vi "10-03-22.vi"() -> ()   [LabVIEW 2015]
uses:
  <vilib>/userdefined/High Color/IMAQdx.ctl
  <vilib>/vision/NI_Vision_Development_Module.lvlib
  <vilib>/vision/driver/NI_Vision_Acquisition_Software.lvlib
panel:
  out "Image 2":T1(plugin-control)
  in  "BCG Values":T2={"Brightness"=171.0, "Contrast"=56.0, "Gamma"=2.0} {"Gamma" min=0.1 max=10 step=0.01 scale=10.0..0.1; "Contrast" min=1 max=89 step=1 scale=30.0..89.0; "Brightness" min=0 max=255 step=1 scale=0.0..255.0}
  out "Processed Image":T1(plugin-control)
  out "error out":errorcluster
  in  "Image Type 2":T3 items=["Grayscale (U8)", "Grayscale (I16)", "Grayscale (SGL)", "Complex (CSG)", "RGB (U32)", "HSL (U32)", "RGB (U64)", "Grayscale (U16)"]
  out "error out 3":errorcluster
  in  "Session In 2":T4
  out "Quantity":i32
  out "Tong K/lg (kg)":dbl
  out "Mass (kg):":dbl
  out "Style":string
  out "Data":string
  out "Found?":bool
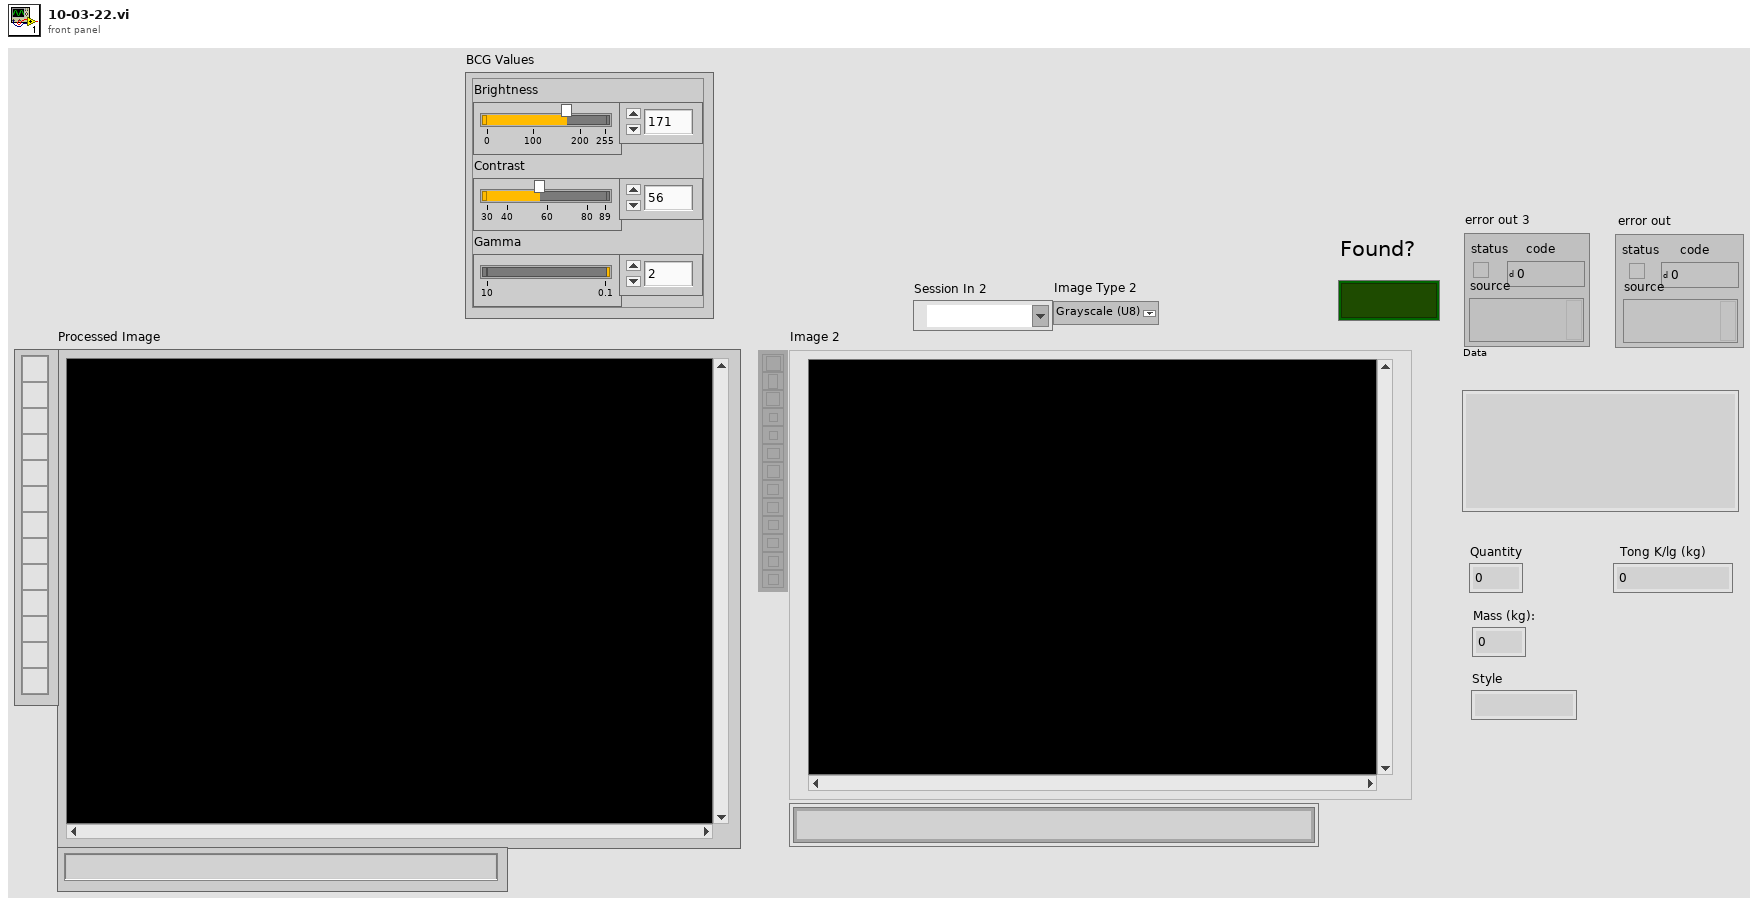
[diagram p1: front panel]
types:
  T1 = typedef "IMAQ Image.ctl" = refnum<image>
  T2 = cluster{"Brightness":sgl, "Contrast":sgl, "Gamma":sgl}
  T3 = typedef "Image Type" = u32
  T4 = typedef "IMAQdx.ctl" = refnum<k21>
  T5 = typedef "QR Code Report.ctl" = cluster{"Found?":bool, "Data":string, "Bounding Box":cluster{"x":sgl, "y":sgl}[], "Errors Corrected":u32, "Dimensions (Rows/Cols)":u32, "Version":u32, "QR Model":T6, "Stream Mode":T7, "Barcode Polarity":T8, "Mirrored?":bool, "Append Stream Position":u32, "Size of Append Stream":u32, "First EAN-128 ID":i32, "First Alternate Language ID":i32, "Append Stream ID":u32, "Minimum Edge Strength":u32, "Demodulation Mode":T9, "Cell Sample Size":T10, "Cell Filter Mode":T11}
  T6 = typedef "QR Code Model Type.ctl" = i32
  T7 = typedef "QR Code Stream Mode Type.ctl" = i32
  T8 = typedef "Data Matrix Polarity.ctl" = i32
  T9 = typedef "Demodulation Mode.ctl" = i32
  T10 = typedef "Cell Sample Size.ctl" = i32
  T11 = typedef "Cell Filter Mode.ctl" = i32
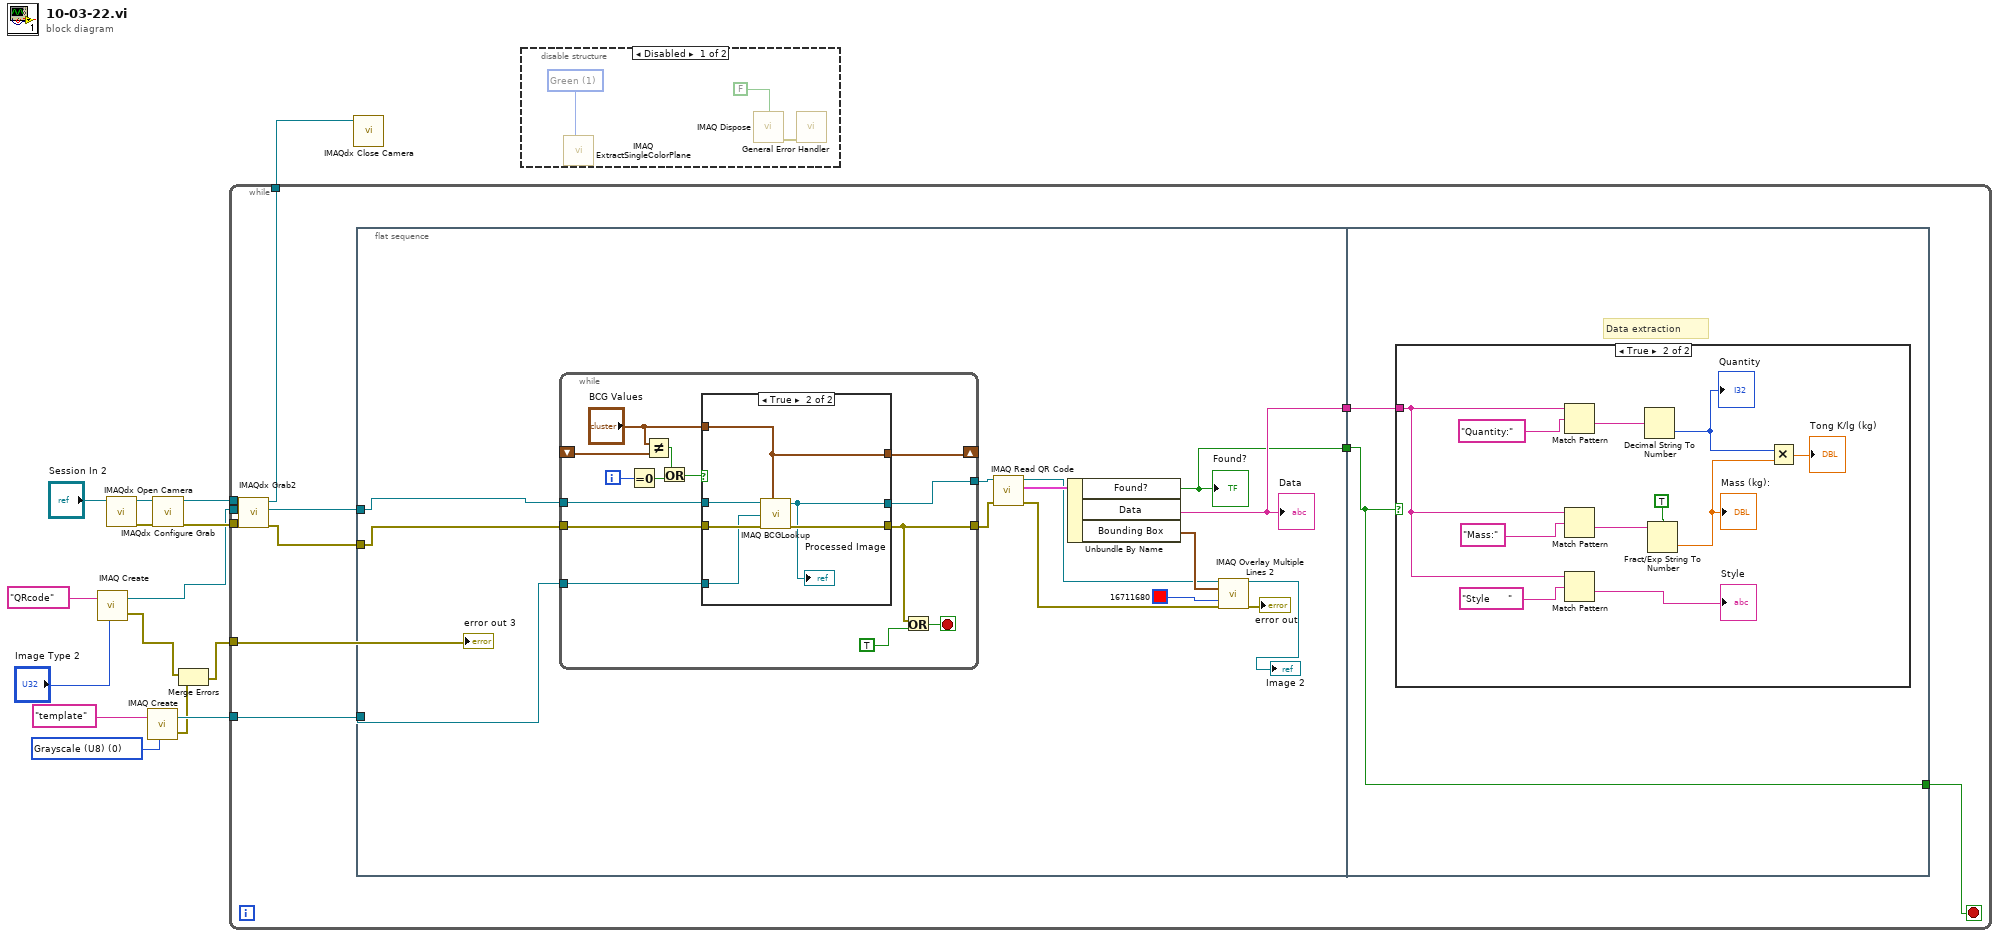
[diagram p0: block diagram]
diagram:
  w9 = T3 0 items=["Grayscale (U8)", "Grayscale (I16)", "Grayscale (SGL)", "Complex (CSG)", "RGB (U32)", "HSL (U32)", "RGB (U64)", "Grayscale (U16)"] ("Image Type")
  n1 = call "IMAQ Create"("Image Name"="QRcode", "Image Type"="Image Type 2") -> ("New Image"=w2:T1, "error out"=w7:errorcluster)  [unwired: 3 in]
  n2 = call <vilib>:"IMAQdx Open Camera.vi"("Session In"="Session In 2") -> ("error out"=w11:errorcluster, "Session Out"=w14:T4)  [unwired: 9 in]
  n3 = call "IMAQ Create"("Image Name"="template", "Image Type"=w9) -> ("New Image"=w8:T1, "error out"=w6:errorcluster)  [unwired: 3 in]
  n4 = call <vilib>:"IMAQdx Configure Grab.vi"("error in"=w11, "Session In"=w14) -> ("error out"=w3:errorcluster, "Session Out"=w4:T4)  [unwired: 8 in]
  n5 = Merge Errors(w7, w6) -> (w5:errorcluster)
  n6 = while {
    tunnel: w8 -> [w24]
    tunnel: w5 -> [w23]
    tunnel: w4 -> [w22]
    tunnel: w3 -> [w21]
    tunnel: w2 -> [w19]
    tunnel: [w16] -> w1
    stop <- w17 stop-if-true
    n7 = call <vilib>:"IMAQdx Grab2.vi"("error in"=w21, "Image In"=w19, "Session In"=w22) -> ("error out"=w20:errorcluster, "Image Out"=w18:T1, "Session Out"=w16:T4)  [unwired: 5 in, 1 out]
    n8 = flat-sequence {
      tunnel: [w36] -> w26
      tunnel: [w30] -> w25
      tunnel: w24 -> [w33]
      tunnel: w20 -> [w27]
      tunnel: w18 -> [w28]
      tunnel: w26 -> [w65]
      tunnel: w25 -> [w64]
      tunnel: [w64] -> w17
      frame #0 {
        n9 = while {
          tunnel: w27 -> [w54]
          tunnel: w28 -> [w53]
          tunnel: w33 -> [w52]
          shift-right: [w51] -> _
          shift-left: _ -> [w50]
          tunnel: [w44] -> w32
          tunnel: [w41] -> w34
          i -> [w48]
          stop <- w43 stop-if-true
          n10 = Equal To 0?(x=w48) -> (x = 0?=w46:bool)
          n11 = Not Equal?(x="BCG Values", y=w50) -> (x != y?=w47:bool)
          n12 = Or(x=w47, y=w46) -> (x .or. y?=w45:bool)
          n13 = case shown="True" w45 {
            tunnel: w54 -> [w57 w63]
            tunnel: w53 -> [_ w62]
            tunnel: "BCG Values" -> [w56 w60]
            tunnel: w52 -> [w55 w61]
            tunnel: [w56 w60] -> w51
            tunnel: [w57 w59] -> w44
            tunnel: [w55 w58] -> w41
            frame False {
            }
            frame True {
              n14 = call "IMAQ BCGLookup"("Image Src"=w62, "BCG Values"=w60, "Image Dst"=w61, "error in (no error)"=w63) -> ("Image Dst Out"=w58:T1, "error out"=w59:errorcluster)  [unwired: 3 in]
              "Processed Image" <- w58
            }
          }
          n15 = Or(x=w44, y=TRUE) -> (x .or. y?=w43:bool)
        }
        n16 = call "IMAQ Read QR Code"("error in (no error)"=w32, "Image"=w34) -> ("error out"=w37:errorcluster, "QR Code Report"=w40:T5, "Image (duplicate)"=w31:T1)  [unwired: 6 in, 1 out]
        n17 = Unbundle By Name(w40) -> ("Found?"=w30:bool, "Data"=w36:string, "Bounding Box"=w39:cluster{"x":sgl, "y":sgl}[])
        "Found?" <- w30
        "Data" <- w36
        n18 = call "IMAQ Overlay Multiple Lines 2"("Image"=w31, "Line End Points"=w39, "Color"=u32 16711680, "error in (no error)"=w37) -> ("Image Out"=→"Image 2":T1, "error out"=→"error out":errorcluster)  [unwired: 10 in]
      }
      frame #1 {
        # "Data extraction"
        n19 = case shown="True" w64 {
          tunnel: w65 -> [_ w66]
          frame False {
          }
          frame True {
            n20 = Match Pattern(string=w66, regular expression="Quantity:") -> (after substring=w68:string)  [unwired: 1 in, 3 out]
            n21 = Match Pattern(string=w66, regular expression="Mass:") -> (after substring=w71:string)  [unwired: 1 in, 3 out]
            n22 = Match Pattern(string=w66, regular expression="Style      ") -> (after substring=→"Style":string)  [unwired: 1 in, 3 out]
            n23 = Decimal String To Number(string=w68) -> (number=w67:i32)  [unwired: 2 in, 1 out]
            "Quantity" <- w67
            n24 = Fract/Exp String To Number(use system decimal point (T)=TRUE, string=w71) -> (number=w74:dbl)  [unwired: 2 in, 1 out]
            "Mass (kg):" <- w74
            n25 = Multiply(x=w67, y=w74) -> (x*y=→"Tong K/lg (kg)":dbl)
          }
        }
      }
    }
    "error out 3" <- w23
  }
  n26 = call <vilib>:"IMAQdx Close Camera.vi"("Session In"=w1) -> ()  [unwired: 10 in, 1 out]
  n27 = disable-structure shown="Disabled" {
    frame Disabled {
      w79 = 1 items=["Red", "Green", "Blue", "Hue", "Saturation", "Luminance", "Value", "Intensity"] ("Color Plane")
      n28 = call "IMAQ ExtractSingleColorPlane"("Color Plane"=w79) -> ()  [unwired: 9 in, 2 out]
      n29 = call "IMAQ Dispose"("All Images? (No)"=FALSE) -> ("error out"=w78:errorcluster)  [unwired: 5 in]
      n30 = call <vilib>:"General Error Handler.vi"("error in (no error)"=w78) -> ()  [unwired: 10 in, 5 out]
    }
    frame Enabled {
    }
  }
